vi "Get_Plot_Scales.vi"(0 "Header In":T1 {"Compression Parameters"."% taper" min=50 max=1000 format="%.2f"; "Compression Parameters"."F2 (MHz)" format="%.3f"; "Compression Parameters"."F1 (MHz)" format="%.3f"; "Scan Settings"."prf (kHz)" format="%.2f"; "Therapy Parameters"."Therapy amplitude (mV)" min=50 max=1000 format="%.2f"; "Therapy Parameters"."Time on (s)" format="%.3f"; "Therapy Parameters"."Theraputic Freq (MHz)" format="%.3f"; "Patient Info"."Race" items=["Am Ind or Alaska", "Asian", "Hawaiian, Pac Isl", "Black or Afr Amer", "White", "more than one race", "unknown"]; "Patient Info"."Ethnicty 2" items=["Hispanic", "Non-Hispanic", "unknown"]; "Patient Info"."LOS" items=["1", "2", "3", "4", "5"]; "Patient Info"."PSA" format="%.1f"; "Scan Info"."delay" format="%.2f"; "Scan Info"."pivot distance" format="%.2f"; "Scan Info"."sector scan angle" format="%.2f"; "Tranducer Info"."bandwidth" format="%.2f"; "Tranducer Info"."center freq" format="%.2f"; "Tranducer Info"."start freq" format="%.2f"}, 5 "Sound Speed modify":i16=1485, 7 "One Way":bool, 9 "Axis scaling":bool, 12 "Optical Spectra":bool) -> (4 "Depth Scale":cluster{"start depth":dbl, "depth interval":dbl}, 6 "Width Scale":cluster{"Start":dbl, "width Interval":dbl})   [LabVIEW 2022 SP3]
uses:
  Header.ctl
panel:
  out "y offset":sgl
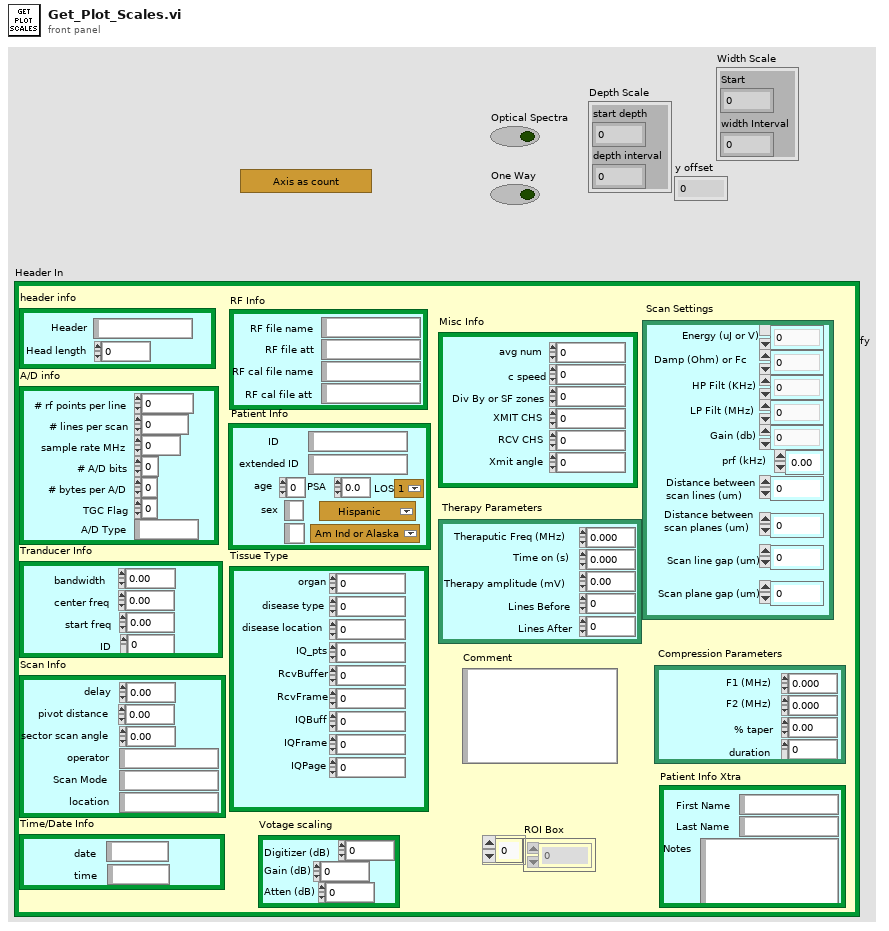
[diagram p1: front panel]
types:
  T1 = typedef "Header.ctl" = cluster{"header info":cluster{"Header":string, "Head length":i16}, "A/D info":cluster{"# rf points per line":u16, "# lines per scan":u16, "sample rate MHz":u16, "# A/D bits":i16, "# bytes per A/D":u16, "TGC Flag":u16, "A/D Type":string}, "Tranducer Info":cluster{"bandwidth":sgl, "center freq":sgl, "start freq":sgl, "ID":i32}, "Scan Info":cluster{"delay":sgl, "pivot distance":sgl, "sector scan angle":sgl, "operator":string, "Scan Mode":string, "location":string}, "Time/Date Info":cluster{"date":string, "time":string}, "RF Info":cluster{"RF file name":string, "RF file att":string, "RF cal file name":string, "RF cal file att":string}, "Patient Info":cluster{"ID":string, "extended ID":string, "age":u16, "sex":string, "previously\nscanned":string, "PSA":sgl, "LOS":u8, "Ethnicty 2":u8, "Race":u8}, "Tissue Type":cluster{"organ":i16, "disease type":i16, "disease location":i16, "IQ_pts":u16, "RcvBuffer":u8, "RcvFrame":u16, "IQBuff":u8, "IQFrame":u16, "IQPage":u8}, "Votage scaling":cluster{"Digitizer (dB)":sgl, "Gain (dB)":sgl, "Atten (dB)":sgl}, "Comment":string, "Misc Info":cluster{"avg num":u16, "c speed":i16, "Div By or SF zones":i16, "XMIT CHS":u8, "RCV CHS":u8, "Xmit angle":sgl}, "Therapy Parameters":cluster{"Theraputic Freq (MHz)":sgl, "Time on (s)":sgl, "Therapy amplitude (mV)":sgl, "Lines Before":u16, "Lines After":u16}, "Scan Settings":cluster{"Energy (uJ or V)":u8, "Damp (Ohm) or Fc":u8, "HP Filt (KHz)":u8, "LP Filt (MHz)":u8, "Gain (db)":u8, "prf (kHz)":sgl, "Distance between\nscan lines (um)":u16, "Distance between\nscan planes (um)":u16, "Scan line gap (um)":sgl, "Scan plane gap (um)":sgl}, "Compression Parameters":cluster{"F1 (MHz)":sgl, "F2 (MHz)":sgl, "% taper":sgl, "duration":sgl}, "Patient Info Xtra":cluster{"First Name":string, "Last Name":string, "Notes":string}, "ROI Box":u16[]}
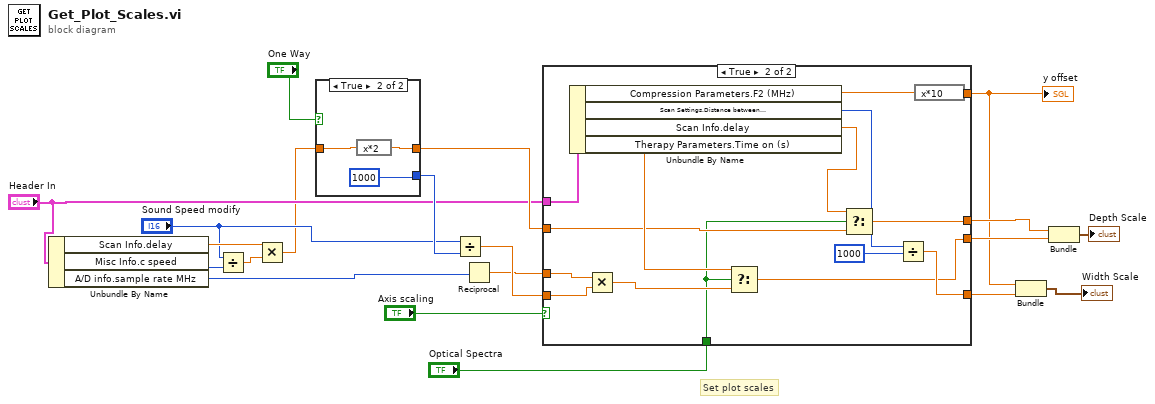
[diagram p0: block diagram]
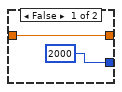
[diagram p2: hidden frame]
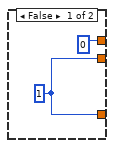
[diagram p3: hidden frame]
diagram:
  # "Set plot scales"
  n1 = Unbundle By Name("Header In") -> ("Scan Info.delay"=w10:sgl, "Misc Info.c speed"=w12:i16, "A/D info.sample rate MHz"=w8:u16)
  n2 = Divide(x="Sound Speed modify", y=w12) -> (x/y=w11:dbl)
  n3 = Multiply(x=w10, y=w11) -> (x*y=w6:dbl)
  n4 = case shown="True" "One Way" {
    tunnel: w6 -> [w22 w24]
    tunnel: [w22 w23] -> w17
    tunnel: [2000 1000] -> w18
    frame False {
    }
    frame True {
      n5 = expression code="x*2"(w24) -> (w23:dbl)
    }
  }
  n6 = Divide(x="Sound Speed modify", y=w18) -> (x/y=w16:dbl)
  n7 = Reciprocal(x=w8) -> (1/x=w15:dbl)
  n8 = case shown="True" "Axis scaling" {
    tunnel: w15 -> [_ w42]
    tunnel: [w27 w35] -> w4
    tunnel: "Header In" -> [_ w41]
    tunnel: [w27 w38] -> w2
    tunnel: [0 w32] -> w3
    tunnel: w17 -> [_ w33]
    tunnel: w16 -> [_ w37]
    tunnel: "Optical Spectra" -> [_ w31]
    tunnel: [_ w28] -> w1
    frame False {
      w27 = 1
    }
    frame True {
      n9 = Unbundle By Name(w41) -> ("Compression Parameters.F2 (MHz)"=w29:sgl, "Scan Settings.Distance between\nscan lines (um)"=w40:u16, "Scan Info.delay"=w30:sgl, "Therapy Parameters.Time on (s)"=w34:sgl)
      n10 = Multiply(x=w42, y=w37) -> (x*y=w36:dbl)
      n11 = Select(t=w34, s=w31, f=w36) -> (s? t:f=w35:dbl)
      n12 = Select(t=w30, s=w31, f=w33) -> (s? t:f=w32:dbl)
      n13 = Divide(x=w40, y=1000) -> (x/y=w38:dbl)
      n14 = expression code="x*10"(w29) -> (w28:sgl)
    }
  }
  "y offset" <- w1
  n15 = Bundle("F2 (MHz)"=w1, w2) -> (→"Width Scale":cluster{"F2 (MHz)":sgl, dbl})  [unwired: 1 in]
  n16 = Bundle("delay"=w3, "Time on (s)"=w4) -> (→"Depth Scale":cluster{"delay":dbl, "Time on (s)":dbl})  [unwired: 1 in]
